vi "Write Header to String Array.vi"(8 "error in (no error)":errorcluster, 11 "Save Image in":refnum<class "Save Image.lvclass">) -> (0 "error out":errorcluster, 3 "Save Image out":refnum<class "Save Image.lvclass">)   [LabVIEW 2018, in "Save Image.lvclass"]
uses:
  Save Image.lvclass
  Save Image.lvclass/Save Image.ctl
  Header/Header.lvclass
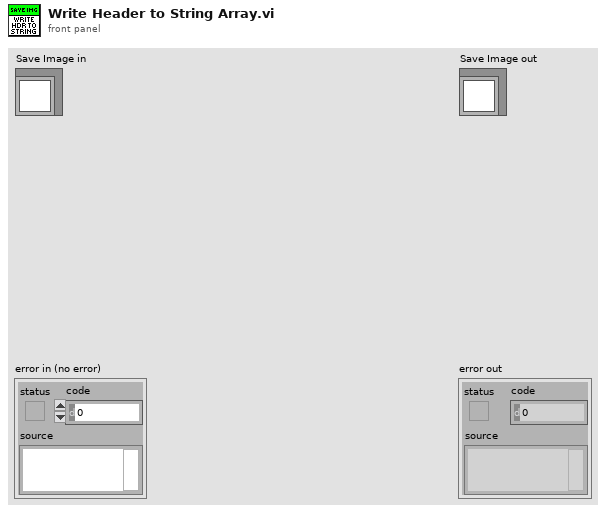
[diagram p1: front panel]
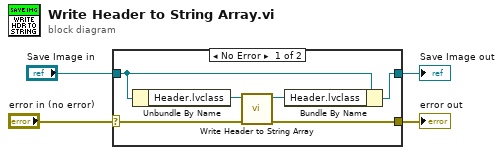
[diagram p0: block diagram]
diagram:
  n1 = case shown="No Error" "error in (no error)" {
    selector: "error in (no error)" -> [w9 w12]
    tunnel: [w10 w12] -> w3
    tunnel: [w6 w11] -> w1
    tunnel: "Save Image in" -> [w7 w11]
    frame No Error {
      n2 = Unbundle By Name(w7) -> ("Header.lvclass"=w8:refnum<class "Header.lvclass">)
      n3 = call "Write Header to String Array.vi"("error in (no error)"=w9, "Header in"=w8) -> ("error out"=w10:errorcluster, "Header out"=w5:refnum<class "Header.lvclass">)  [unwired: 8 in]
      n4 = Bundle By Name(cluster=w7, "Header.lvclass"=w5) -> (w6:refnum<class "Save Image.lvclass">)
    }
    frame Error {
    }
  }
  "error out" <- w3
  "Save Image out" <- w1
